vi "set_As_Liq0.vi"(7 "As_Liq Flow":dbl, 8 "As_Liq Remote":bool, 9 "As_Liq Run":bool, 10 "As_Liq Bubbler":bool, 11 "As_Liq Active":bool) -> ()   [LabVIEW 2011]
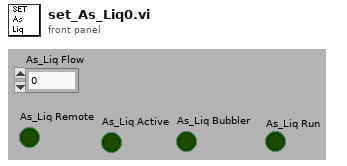
[diagram p1: front panel]
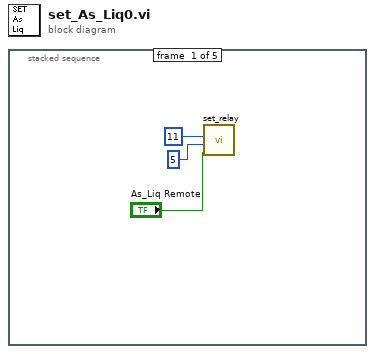
[diagram p0: block diagram]
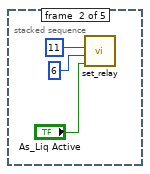
[diagram p2: hidden frame]
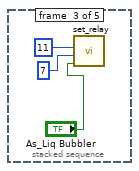
[diagram p3: hidden frame]
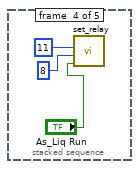
[diagram p4: hidden frame]
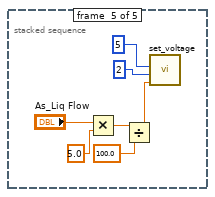
[diagram p5: hidden frame]
diagram:
  n1 = stacked-sequence {
    frame #0 {
      n2 = call "set_relay.vi"("Slot"=11, "Relay"=5, "Relay Status"="As_Liq Remote") -> ()  [unwired: 3 out]
    }
    frame #1 {
      n3 = call "set_relay.vi"("Slot"=11, "Relay"=6, "Relay Status"="As_Liq Active") -> ()  [unwired: 3 out]
    }
    frame #2 {
      n4 = call "set_relay.vi"("Slot"=11, "Relay"=7, "Relay Status"="As_Liq Bubbler") -> ()  [unwired: 3 out]
    }
    frame #3 {
      n5 = call "set_relay.vi"("Slot"=11, "Relay"=8, "Relay Status"="As_Liq Run") -> ()  [unwired: 3 out]
    }
    frame #4 {
      n6 = Multiply(x="As_Liq Flow", y=5.0) -> (x*y=w16:dbl)
      n7 = Divide(x=w16, y=100.0) -> (x/y=w18:dbl)
      n8 = call "set_voltage.vi"("Voltage"=w18, "Channel"=2, "Slot"=5) -> ()  [unwired: 1 in, 1 out]
    }
  }
